vi "Get Control Ref By Class Name.vi"(8 "error in (no error)":errorcluster, 10 "Control Class":string(combo), 11 "Setting View in":refnum<class "Setting View.lvclass">) -> (0 "error out":errorcluster, 1 "refs":refnum<vi>[](array[refnum]), 3 "Setting View out":refnum<class "Setting View.lvclass">)   [LabVIEW 2020, in "[V]Setting View.lvlib" / "Setting View.lvclass"]
uses:
  Setting View.lvclass
  Depden On/Abstruct View/Abstruct View/Abstruct View.lvclass/Abstruct View.ctl
  Depden On/Abstruct View/Abstruct View/Data Accessors/Read Core VI.vi
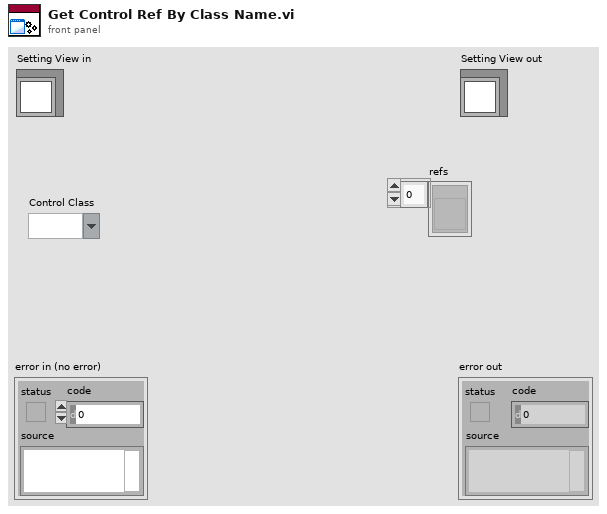
[diagram p1: front panel]
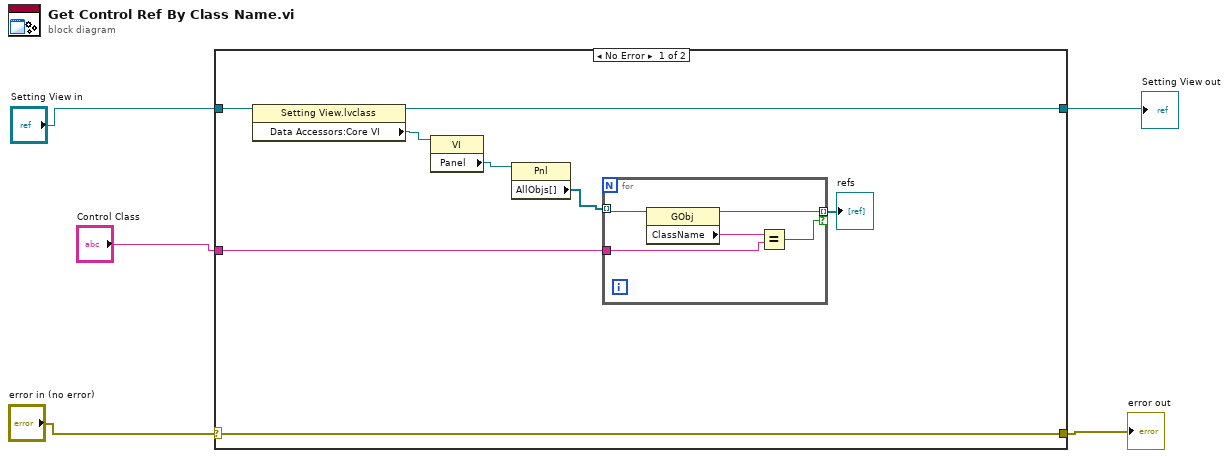
[diagram p0: block diagram]
diagram:
  n1 = case shown="No Error" "error in (no error)" {
    selector: "error in (no error)" -> [w13 w20]
    tunnel: [w13 w20] -> w2
    tunnel: [w11 w19] -> w4
    tunnel: "Setting View in" -> [w12 w19]
    tunnel: "Control Class" -> [w6 _]
    frame No Error {
      n2 = property class="Setting View.lvclass"(reference=w12) -> (reference out=w11:refnum<class "Setting View.lvclass">, "Data Accessors:Core VI"=w8:refnum<vi>)  [unwired: 1 in, 1 out]
      n3 = property class="VI"(reference=w8) -> ("Panel"=w10:refnum<vi>)  [unwired: 1 in, 2 out]
      n4 = property class="Pnl"(reference=w10) -> ("AllObjs[]"=w9:refnum<vi>[])  [unwired: 1 in, 2 out]
      n5 = for {
        tunnel: w9 -> [w18] mode=indexing
        tunnel: [w16] -> w7 mode=indexing if=w15
        tunnel: w6 -> [w14]
        n6 = property class="GObj"(reference=w18) -> (reference out=w16:refnum<vi>, "ClassName"=w17:string)  [unwired: 1 in, 1 out]
        n7 = Equal?(x=w17, y=w14) -> (x = y?=w15:bool)
      }
      "refs" <- w7
    }
    frame Error {
    }
  }
  "error out" <- w2
  "Setting View out" <- w4
